vi "TP 1.1.vi"() -> ()   [LabVIEW 2013]
panel:
  out "Cadena":string
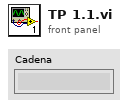
[diagram p1: front panel]
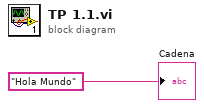
[diagram p0: block diagram]
diagram:
  "Cadena" <- "Hola Mundo"
